vi "Peak Filtering.vi"(8 "Tau_+":dbl, 9 "Tau_sigma":dbl, 10 "Salience Peaks":dbl[](array[numeric])) -> (1 "S-":dbl[](array[numeric]), 2 "S+":dbl[](array[numeric]))   [LabVIEW 2014]
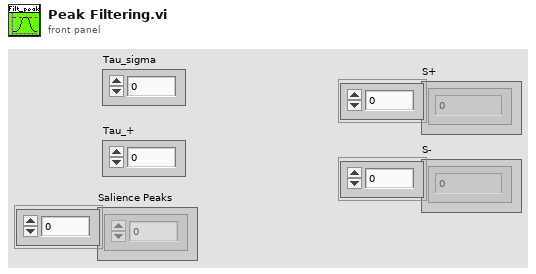
[diagram p1: front panel]
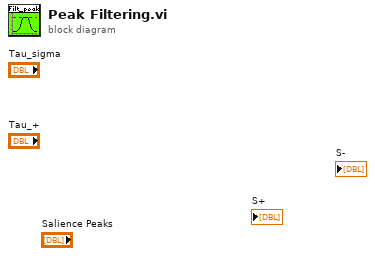
[diagram p0: block diagram]
diagram:
